vi "Log_channels.vi"(5 "History (min)":dbl=5.0 min=5.0 max=70.0 format="%.1f") -> ()   [LabVIEW 2010]
uses:
  Sub VIs/ADAM Controls/Search_mode.ctl
panel:
  out "Last wrote to file":string
  in  "Logging on":bool
  in  "Data Filename":path
  out "Last Updated":string
  in  "stop":bool
  in  "Mode":T1(ring)
  in  "Selector 1":i32[](listbox)
  out "Plot 1":cluster{dbl[], "Output array":dbl[]}[](graph)
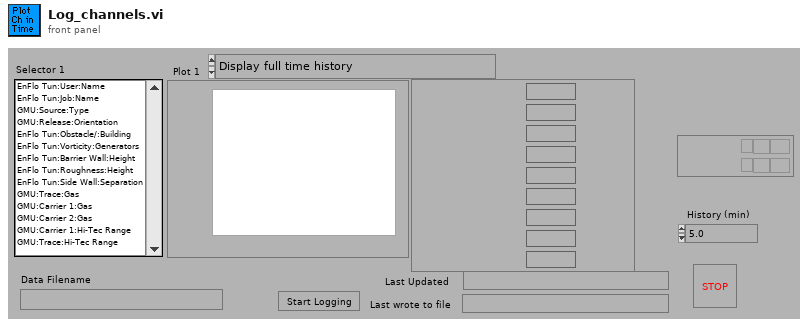
[diagram p1: front panel]
types:
  T1 = enum16{"Display full time history", "Display data over specified period"}
  T2 = typedef "Search_mode.ctl" = enum16{"Between times", "All Times"}
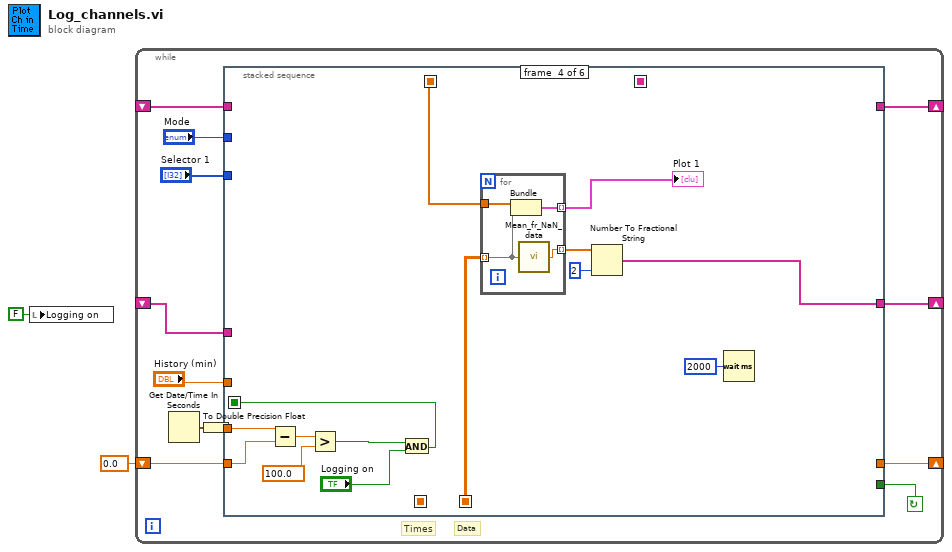
[diagram p0: block diagram]
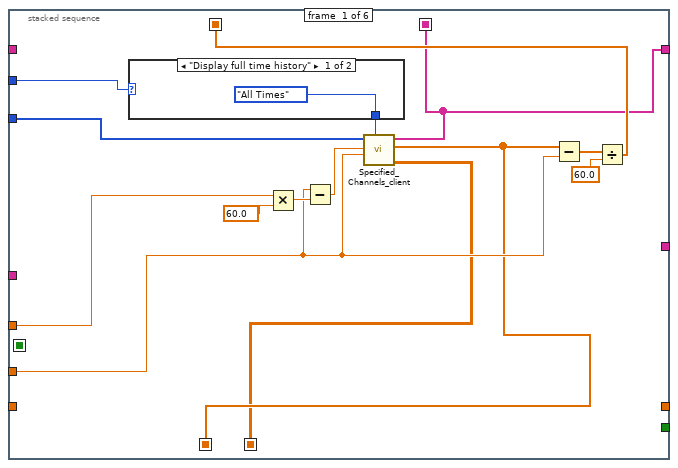
[diagram p2: hidden frame]
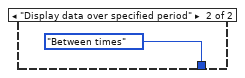
[diagram p3: hidden frame]
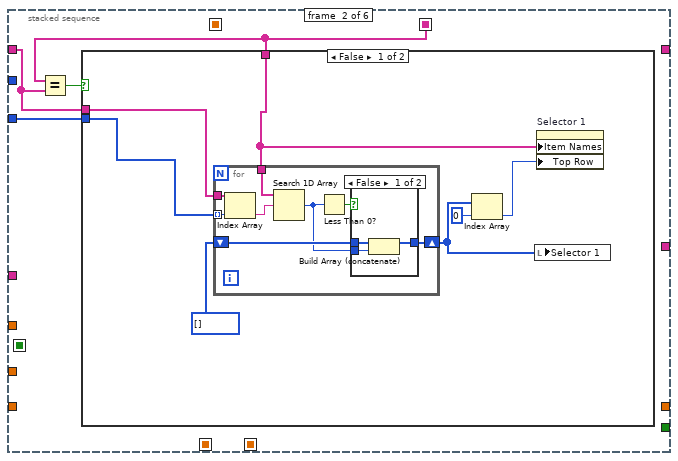
[diagram p4: hidden frame]
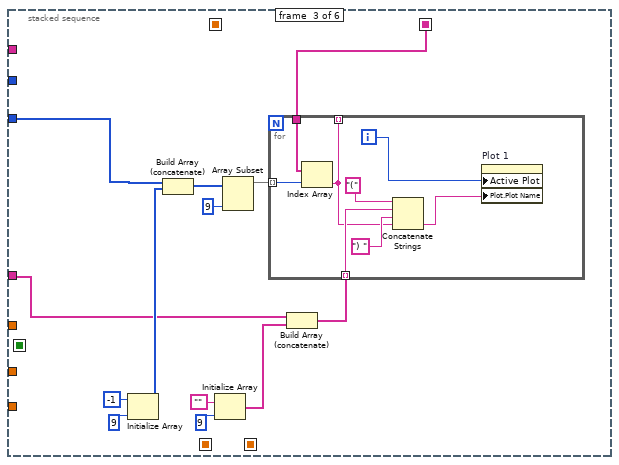
[diagram p7: hidden frame]
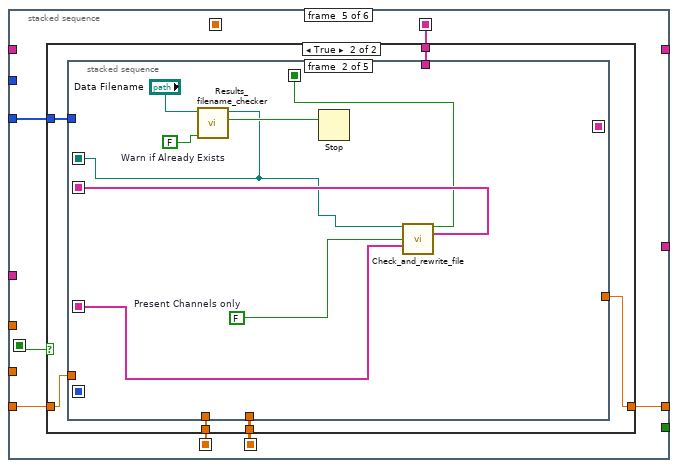
[diagram p8: hidden frame]
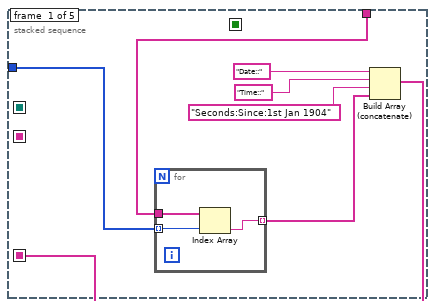
[diagram p10: hidden frame]
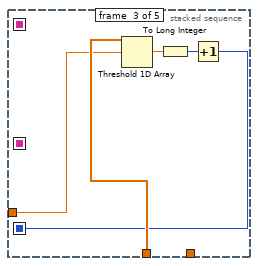
[diagram p11: hidden frame]
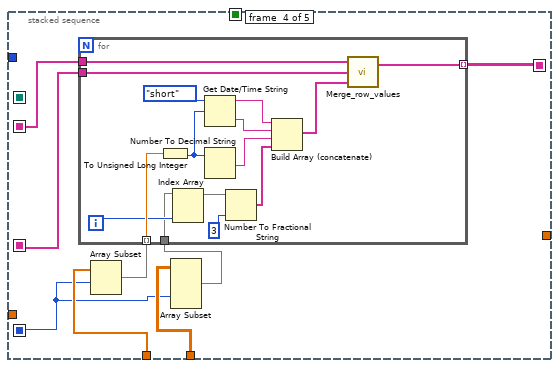
[diagram p12: hidden frame]
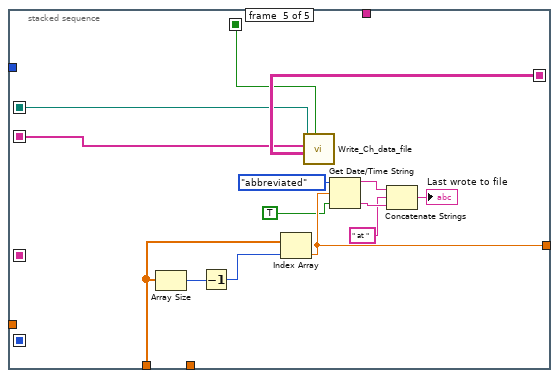
[diagram p13: hidden frame]
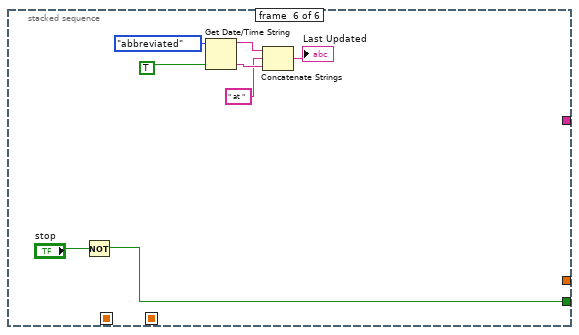
[diagram p14: hidden frame]
diagram:
  n1 = local write "Logging on"(FALSE ("Logging on")) -> ()
  n2 = while {
    shift-left: 0.0 -> [w5]
    shift-right: [w4] -> _
    shift-left: _ -> [w11]
    shift-right: [w12] -> _
    shift-left: _ -> [w13]
    shift-right: [w14] -> _
    stop <- w7 continue-if-true
    # "Data"
    # "Times"
    n3 = Get Date/Time In Seconds() -> (seconds since 1Jan1904=w3:timestamp)
    n4 = To Double Precision Float(number=w3) -> (double precision float=w6:dbl)
    n5 = stacked-sequence {
      seq-local: [w22 _ _ _ _ _] -> [_ _ _ w87 _ _]
      seq-local: [w15 _ _ _ _ _] -> [_ _ _ w76 w95 _]
      seq-local: [w21 _ _ _ _ _] -> [_ w32 w64 _ w93 _]
      seq-local: [w16 _ _ _ _ _] -> [_ _ _ _ w96 _]
      seq-local: [_ _ _ w77 _ _] -> [_ _ _ _ w99 _]
      tunnel: [_ _ _ w88 _ _] -> w14
      tunnel: w13 -> [_ _ w54 _ _ _]
      tunnel: [w21 _ _ _ _ _] -> w12
      tunnel: w11 -> [_ w33 _ _ _ _]
      tunnel: "Selector 1" -> [w18 w31 w63 _ w94 _]
      tunnel: "Mode" -> [w20 _ _ _ _ _]
      tunnel: "History (min)" -> [w19 _ _ _ _ _]
      tunnel: [_ _ _ _ _ w173] -> w7
      tunnel: w6 -> [w17 _ _ w75 _ _]
      tunnel: w5 -> [_ _ _ w82 w97 _]
      tunnel: [_ _ _ _ w98 _] -> w4
      frame #0 {
        n6 = case shown="\"Display full time history\"" w20 {
          tunnel: [Search_mode."All Times" ("Mode") enum16{"Between times", "All Times"}."Between times" ("Mode")] -> w25
          frame "Display full time history" {
          }
          frame "Display data over specified period" {
          }
        }
        n7 = Multiply(x=w19, y=60.0) -> (x*y=w27:dbl)
        n8 = Subtract(x=w17, y=w27) -> (x-y=w26:dbl)
        n9 = call "Specified_Channels_client.vi"("Mode"=w25, "End time"=w17, "Start time"=w26, "ADAM Index array"=w18) -> ("Output array"=w15:dbl[][], "Centre Times"=w16:dbl[], "All Active Ch Names"=w21:string[])  [unwired: 1 in, 4 out]
        n10 = Subtract(x=w16, y=w17) -> (x-y=w24:dbl[])
        n11 = Divide(x=w24, y=60.0) -> (x/y=w22:dbl[])
      }
      frame #1 {
        n12 = Equal?(x=w32, y=w33) -> (x = y?=w34:bool)
        n13 = case shown="False" w34 {
          tunnel: w33 -> [w41 _]
          tunnel: w32 -> [w40 _]
          tunnel: w31 -> [w39 _]
          frame False {
            n14 = for {
              tunnel: w39 -> [w49] mode=indexing
              tunnel: w41 -> [w48]
              tunnel: w40 -> [w46]
              shift-right: [w42] -> w36
              shift-left: i32[] [] -> [w44]
              n15 = Index Array(array=w48, index=w49) -> (element=w47:string)
              n16 = Search 1D Array(1D array=w46, element=w47) -> (index of element=w43:i32)  [unwired: 1 out]
              n17 = Less Than 0?(x=w43) -> (x < 0?=w45:bool)
              n18 = case shown="False" w45 {
                tunnel: w44 -> [w52 w53]
                tunnel: w43 -> [w51 _]
                tunnel: [w50 w53] -> w42
                frame False {
                  n19 = Build Array (concatenate)(w52, w51) -> (w50:i32[])
                }
                frame True {
                }
              }
            }
            n20 = Index Array(array=w36, index=0) -> (element=w35:i32)
            n21 = local write "Selector 1"(w36) -> ()
            n22 = property on="Selector 1" class="LstBox (strict)"("Item Names"=w40, "Top Row"=w35) -> ()  [unwired: 2 in, 2 out]
          }
          frame True {
          }
        }
      }
      frame #2 {
        n23 = Initialize Array(-1, 9) -> (w60:i32[])
        n24 = Build Array (concatenate)(w63, w60) -> (w58:i32[])
        n25 = Initialize Array("", 9) -> (w59:string[])
        n26 = Array Subset(array=w58, length=9) -> (w57:i32[])  [unwired: 1 in]
        n27 = Build Array (concatenate)(w54, w59) -> (w55:string[])
        n28 = for {
          tunnel: w64 -> [w70]
          tunnel: w55 -> [w69] mode=indexing
          tunnel: w57 -> [w68] mode=indexing
          tunnel: [w67] -> _ mode=indexing
          i -> [w71]
          n29 = Index Array(array=w70, index=w68) -> (element=w67:string)
          n30 = Concatenate Strings("(", w69, ") ", w67) -> (w74:string)
          n31 = property on="Plot 1" class="XYGraph (strict)"("Active Plot"=w71, "Plot.Plot Name"=w74) -> ()  [unwired: 2 in, 2 out]
        }
      }
      frame #3 {
        n32 = Subtract(x=w75, y=w82) -> (x-y=w81:dbl)
        n33 = Greater?(x=w81, y=100.0) -> (0:w79:bool)
        n34 = And(x=w79, y="Logging on") -> (x .and. y?=w77:bool)
        n35 = for {
          tunnel: w76 -> [w91] mode=indexing
          tunnel: [w92] -> w84 mode=indexing
          tunnel: [w90] -> w85 mode=indexing
          tunnel: w87 -> [w89]
          n36 = Bundle(w89, "Output array"=w91) -> (w92:cluster{dbl[], "Output array":dbl[]})  [unwired: 1 out]
          n37 = call "Mean_fr_NaN_data.vi"("Data"=w91) -> ("Mean value"=w90:dbl)
        }
        "Plot 1" <- w84
        n38 = Number To Fractional String(number=w85, precision (6)=i16 2) -> (F-format string=w88:string[])  [unwired: 2 out]
        n39 = Wait (ms)(milliseconds to wait=u32 2000 ("milliseconds to Wait")) -> ()  [unwired: 1 out]
      }
      frame #4 {
        n40 = case shown="True" w99 {
          tunnel: [w100 w105] -> w98
          tunnel: w97 -> [w100 w103]
          tunnel: w96 -> [_ w106]
          tunnel: w95 -> [_ w104]
          tunnel: w94 -> [_ w102]
          tunnel: w93 -> [_ w101]
          frame False {
          }
          frame True {
            n41 = stacked-sequence {
              seq-local: [_ w117 _ _ _] -> [_ _ _ _ w161]
              seq-local: [_ w122 _ _ _] -> [_ _ _ w137 w162]
              seq-local: [_ w121 _ _ _] -> [_ _ _ _ w160]
              seq-local: [w107 _ _ _ _] -> [_ w119 _ w136 _]
              seq-local: [_ _ w125 _ _] -> [_ _ _ w131 _]
              seq-local: [_ _ _ w132 _] -> [_ _ _ _ w163]
              tunnel: w106 -> [_ _ w129 w135 w166]
              tunnel: [_ _ _ _ w155] -> w105
              tunnel: w104 -> [_ _ _ w133 _]
              tunnel: w103 -> [_ _ w127 _ _]
              tunnel: w102 -> [w110 _ _ _ _]
              tunnel: w101 -> [w109 _ _ _ _]
              frame #0 {
                n42 = for {
                  tunnel: w110 -> [w116] mode=indexing
                  tunnel: w109 -> [w115]
                  tunnel: [w114] -> w108 mode=indexing
                  n43 = Index Array(array=w115, index=w116) -> (element=w114:string)
                }
                n44 = Build Array (concatenate)("Date::", "Time::", "Seconds:Since:1st Jan 1904", w108) -> (w107:string[])
              }
              frame #1 {
                w123 = FALSE  # Present Channels only
                w124 = FALSE  # Warn if Already Exists
                n45 = call "Results_filename_checker.vi"("Warn if Already Exists"=w124, "Results file"="Data Filename") -> ("cancelled"=w118:bool, "Results file output"=w117:path)  [unwired: 3 in, 2 out]
                n46 = Stop(stop? (T)=w118) -> ()
                n47 = call "Check_and_rewrite_file.vi"("Filename"=w117, "Present Channels only"=w123, "Present Channels"=w119) -> ("exists?"=w121:bool, "Merged Channels"=w122:string[])  [unwired: 1 in, 10 out]
              }
              frame #2 {
                n48 = Threshold 1D Array(2:w127, 3:w129) -> (0:w128:dbl)  [unwired: 1 out]
                n49 = To Long Integer(number=w128) -> (32bit integer=w126:i32)
                n50 = Increment(x=w126) -> (x+1=w125:i32)
              }
              frame #3 {
                n51 = Array Subset(array=w135, index=w131) -> (w134:dbl[])  [unwired: 1 in]
                n52 = Array Subset(array=w133, index (col)=w131) -> (w130:dbl[][])  [unwired: 3 in]
                n53 = for {
                  tunnel: w134 -> [w152] mode=indexing
                  tunnel: w137 -> [w149]
                  tunnel: w136 -> [w145]
                  tunnel: [w142] -> w132 mode=indexing
                  tunnel: w130 -> [w140]
                  i -> [w141]
                  n54 = To Unsigned Long Integer(number=w152) -> (unsigned 32bit integer=w151:u32)
                  n55 = Index Array(array=w140, index (col)=w141) -> (element=w139:dbl[])  [unwired: 1 in]
                  n56 = Get Date/Time String(date format (0)=enum16{"short", "long", "abbreviated"}."short", seconds (now)=w151) -> (date string=w148:string, time string=w147:string)  [unwired: 1 out]
                  n57 = Number To Decimal String(number=w151) -> (decimal integer string=w146:string)  [unwired: 1 out]
                  n58 = Number To Fractional String(number=w139, precision (6)=i16 3) -> (F-format string=w143:string[])  [unwired: 2 out]
                  n59 = Build Array (concatenate)(w148, w147, w146, w143) -> (w144:string[])
                  n60 = call "Merge_row_values.vi"("Present Row values"=w144, "Present Channels"=w145, "Desired Channels"=w149) -> ("Desired Row values"=w142:string[])  [unwired: 1 out]
                }
              }
              frame #4 {
                n61 = Array Size(array=w166) -> (size(s)=w165:i32)
                n62 = Decrement(x=w165) -> (x-1=w164:i32)
                n63 = Index Array(array=w166, index=w164) -> (element=w155:dbl)
                n64 = call "Write_Ch_data_file.vi"("exists?"=w160, "Channel Values"=w163, "Channel names"=w162, "Filename"=w161) -> ()  [unwired: 4 in, 4 out]
                n65 = Get Date/Time String(date format (0)=enum16{"short", "long", "abbreviated"}."abbreviated", seconds (now)=w155, want seconds? (F)=TRUE) -> (date string=w158:string, time string=w157:string)
                n66 = Concatenate Strings(w158, " at " ("Substring"), w157) -> (→"Last wrote to file":string)
              }
            }
          }
        }
      }
      frame #5 {
        n67 = Not(x="stop") -> (.not. x?=w173:bool)
        n68 = Get Date/Time String(date format (0)=enum16{"short", "long", "abbreviated"}."abbreviated", want seconds? (F)=TRUE) -> (date string=w171:string, time string=w169:string)  [unwired: 1 out]
        n69 = Concatenate Strings(w171, " at " ("Substring"), w169) -> (→"Last Updated":string)
      }
    }
  }
